vi "FFT_based_prediction_Computationtime.vi"() -> ()   [LabVIEW 2020]
uses:
  <vilib>/Utility/file.llb/Read Delimited Spreadsheet (DBL).vi
panel:
  out "x-y":u32
  out "Time vs Acceleration graph(whole data)  2":cluster{"all rows":dbl[], "all rows":dbl[]}(graph)
  out "Acceleration 3":dbl[](array[numeric])
  out "time 3":dbl[](array[numeric])
  out "array w/ subset deleted 3":dbl[][](array[numeric])
  out "Input vs prediction (zoomed) 2":dbl[][](graph)
  out "truth vs prediction vs error 2":dbl[][](graph)
  out "Input vs prediction  2":dbl[][](graph)
  out "Time vs Acceleration ( Input learning length) 2":cluster{dbl[], dbl[]}[](graph)
  out "magnitude 4":dbl[](array[numeric])
  out "phase 4":dbl[](array[numeric])
  out "ploted signal from each selected frequency 3":dbl[][](graph)
  out "df (Hz) 3":dbl
  out "size(s) 3":i32
  out "xf (frequency) 3":dbl[](array[numeric])
  out "Frequency Interval: delta(f) 3":dbl
  out "Spectrum plot 3":cluster{i32, dbl, "spectrum out":dbl[]}(graph)
  out "truth vs prediction  2":dbl[][](graph)
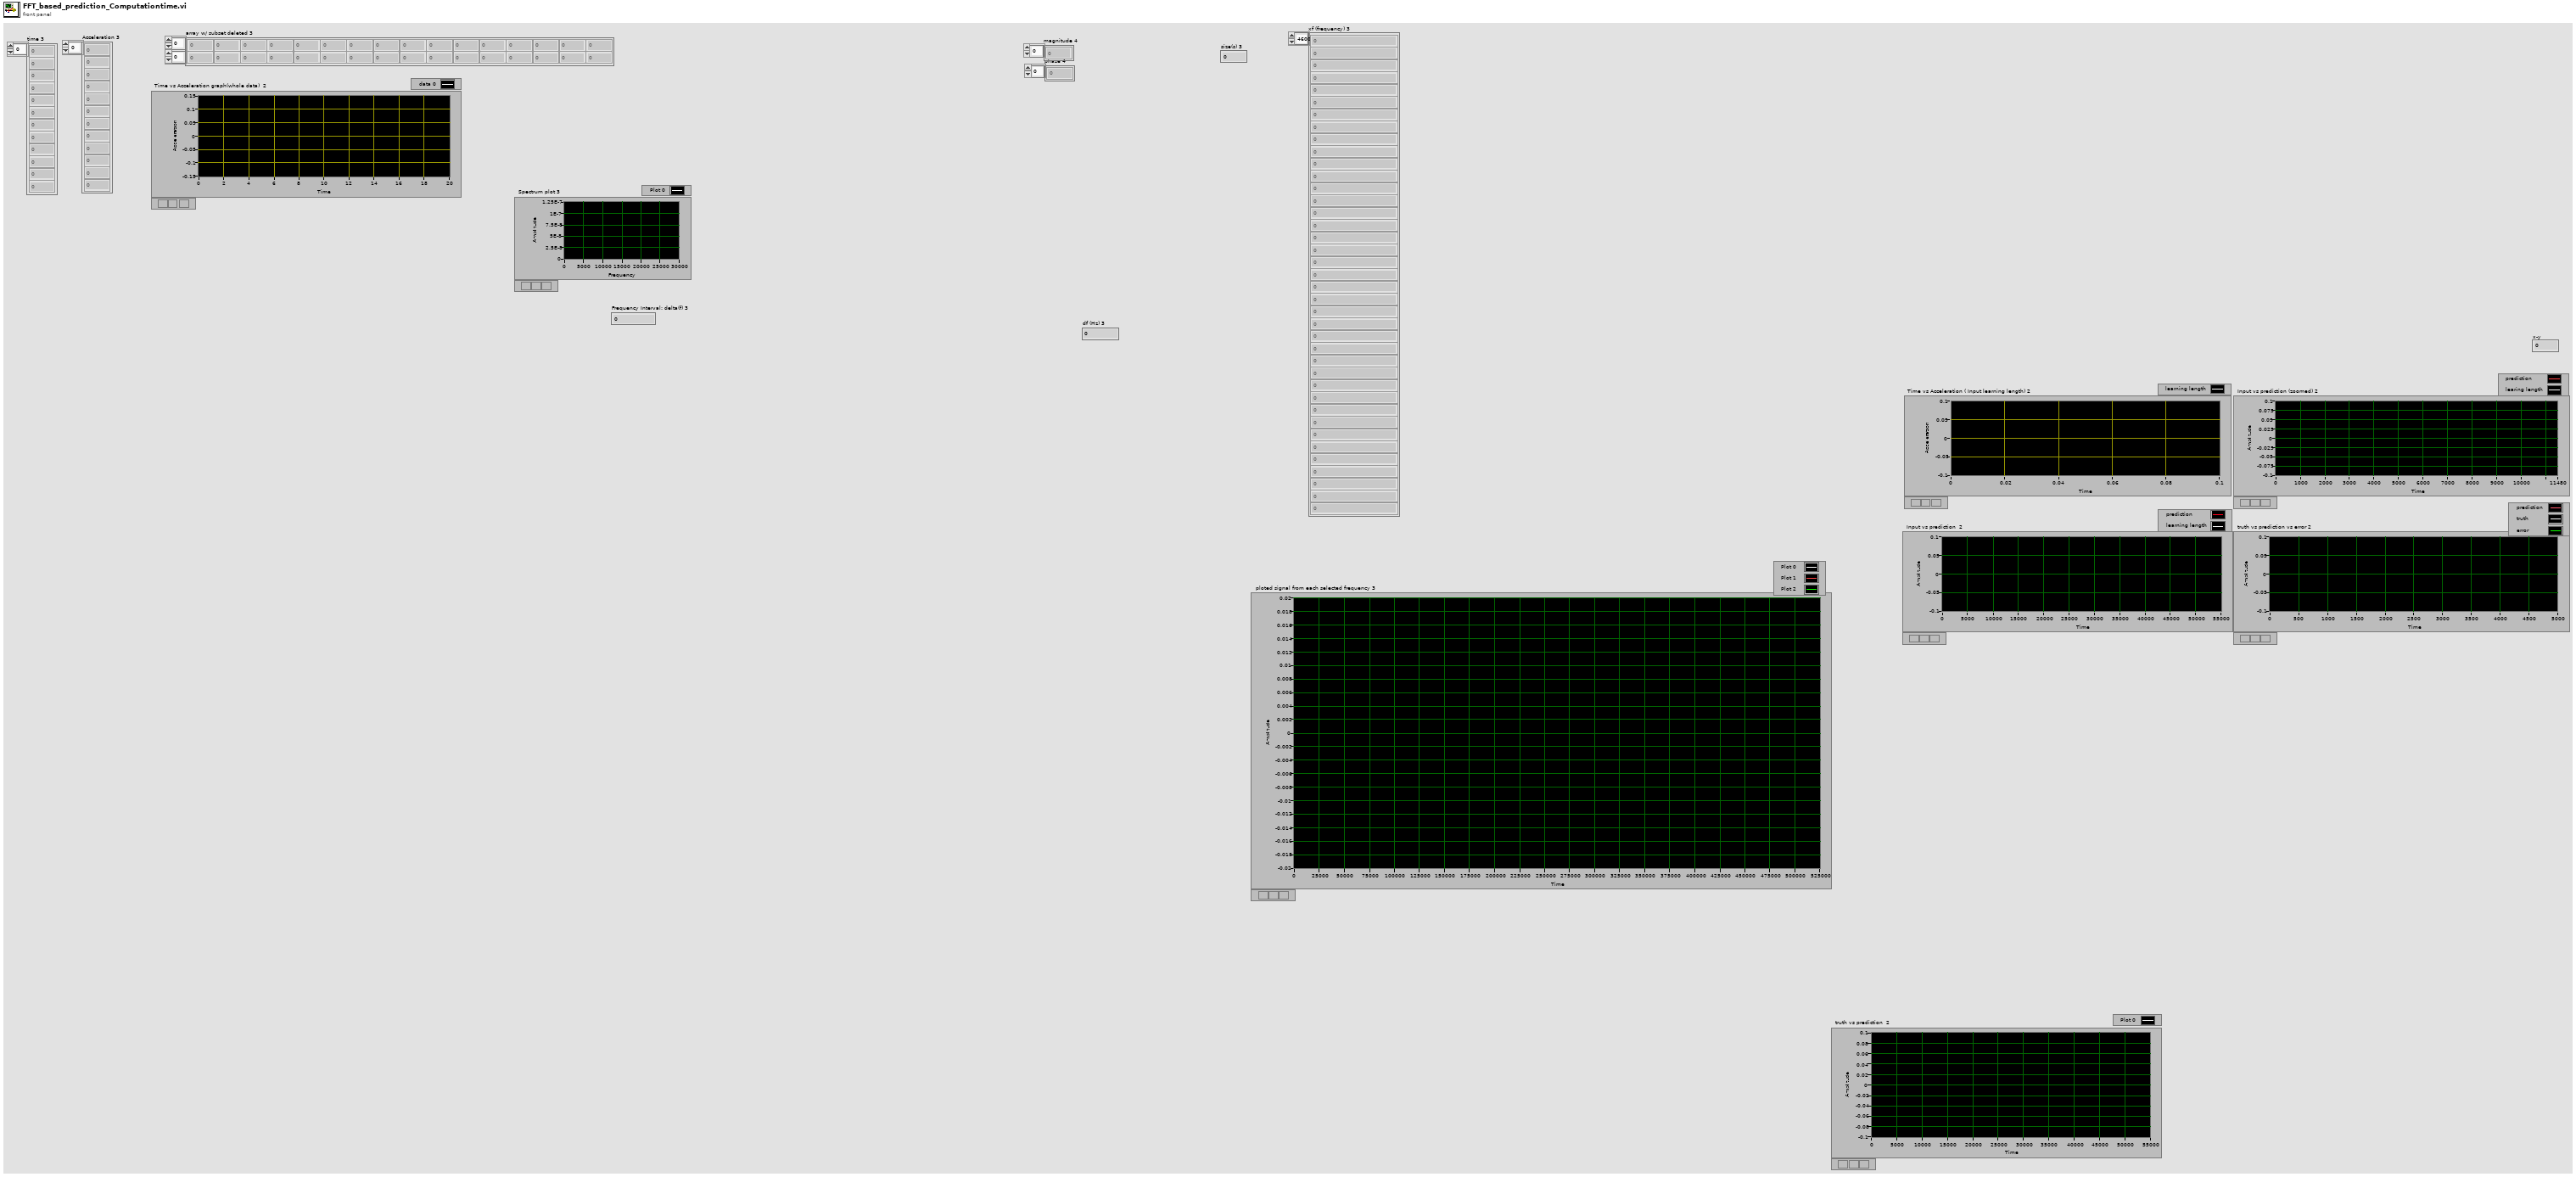
[diagram p1: front panel]
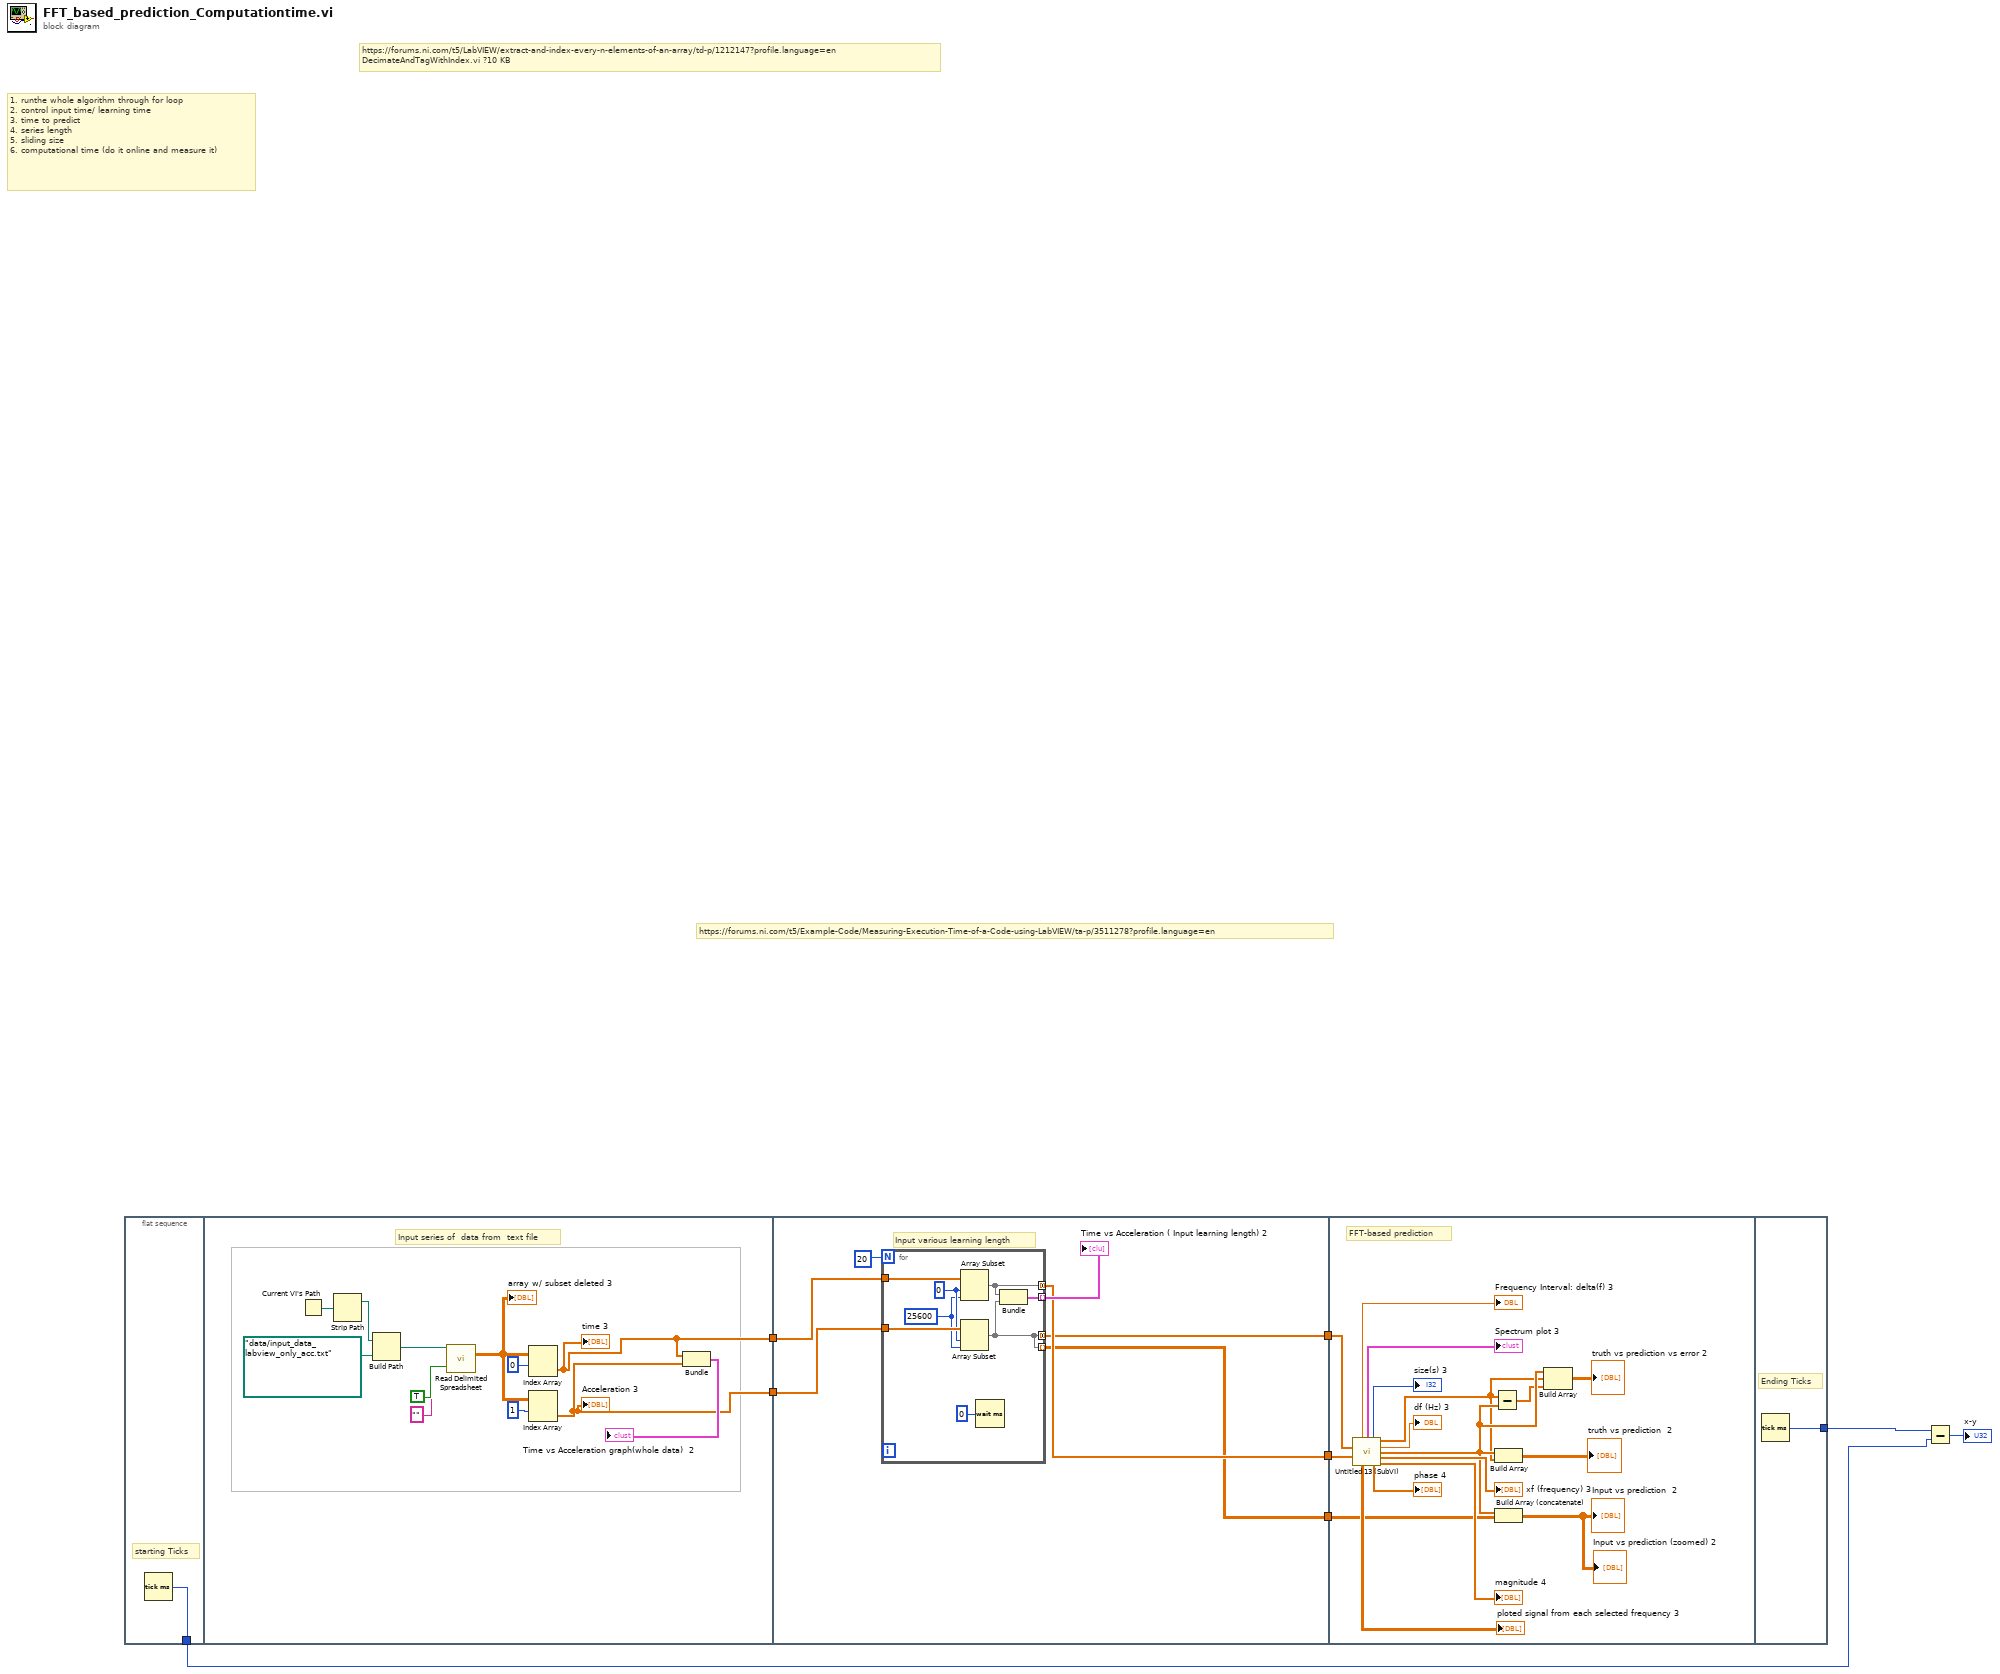
[diagram p0: block diagram]
diagram:
  # "https://forums.ni.com/t5/Example-Code/Measuring-Execution-Time-of-a-Code-using-LabVIEW/ta-p/3511278?profile.language=en"
  # "1. runthe whole algorithm through for loop \n2. control input time/ learning time\n3. time to predict\n4. series length\n5. sliding size\n6. computational time (do it online and measure it)"
  # "https://forums.ni.com/t5/LabVIEW/extract-and-index-every-n-elements-of-an-array/td-p/1212147?profile.language=en\nDecimateAndTagWithIndex.vi ?10 KB"
  n1 = flat-sequence {
    tunnel: [w9] -> w1
    tunnel: [w11] -> w8
    tunnel: [w10] -> w7
    tunnel: w8 -> [w27]
    tunnel: w7 -> [w26]
    tunnel: [w24] -> w6
    tunnel: [w23] -> w5
    tunnel: [w22] -> w4
    tunnel: w6 -> [w39]
    tunnel: w5 -> [w38]
    tunnel: w4 -> [w37]
    tunnel: [w54] -> w3
    frame #0 {
      # "starting Ticks"
      n2 = Tick Count (ms)() -> (millisecond timer value=w9:u32)
    }
    frame #1 {
      # "Input series of  data from  text file"
      n3 = Current VI's Path() -> (path=w19:path)
      n4 = Strip Path(path=w19) -> (stripped path=w20:path)  [unwired: 1 out]
      n5 = Build Path(base path=w20, name or relative path=path "data/input_data_labview_only_acc.txt") -> (appended path=w21:path)
      n6 = call-poly <vilib>:"Read Delimited Spreadsheet.vi"("file path (dialog if empty)"=w21, "transpose? (F)"=TRUE, "delimiter (\\t)"="" ("delimiter (\\t)")) -> ("all rows"=w18:dbl[][])  [unwired: 7 in, 5 out]
      "array w/ subset deleted 3" <- w18
      n7 = Index Array(array=w18, index (row)=0) -> (element=w11:dbl[])  [unwired: 1 in]
      "time 3" <- w11
      n8 = Index Array(array=w18, index (row)=1) -> (element=w10:dbl[])  [unwired: 1 in]
      "Acceleration 3" <- w10
      n9 = Bundle("all rows"=w11, "all rows"=w10) -> (→"Time vs Acceleration graph(whole data)  2":cluster{"all rows":dbl[], "all rows":dbl[]})  [unwired: 1 in]
    }
    frame #2 {
      # "Input various learning length"
      n10 = for {
        N: 20 -> [_]
        tunnel: w27 -> [w36]
        tunnel: [w33] -> w24 mode=concatenating
        tunnel: w26 -> [w35]
        tunnel: [w31] -> w23 mode=concatenating
        tunnel: [w32] -> w25 mode=indexing
        tunnel: [w31] -> w22 mode=indexing
        w34 = 0
        w30 = 25600 ("length")
        n11 = Array Subset(array=w36, index=w34, length=w30) -> (w33:dbl[])
        n12 = Array Subset(array=w35, index=w34, length=w30) -> (w31:dbl[])
        n13 = Wait (ms)(milliseconds to wait=u32 0) -> ()  [unwired: 1 out]
        n14 = Bundle(w33, w31) -> (w32:cluster{dbl[], dbl[]})  [unwired: 1 in]
      }
      "Time vs Acceleration ( Input learning length) 2" <- w25
    }
    frame #3 {
      # "FFT-based prediction"
      n15 = call "Untitled 13 (SubVI).vi"("time"=w39, "acceleration"=w38) -> ("Frequency Interval: delta(f)"=→"Frequency Interval: delta(f) 3":dbl, "Spectrum plot"=→"Spectrum plot 3":cluster{i32, dbl, "spectrum out":dbl[]}, "size(s)"=→"size(s) 3":i32, "all rows"=w43:dbl[], "df (Hz)"=→"df (Hz) 3":dbl, "Array"=w44:dbl[], "xf (frequency)"=→"xf (frequency) 3":dbl[], "ploted signal from each selected frequency"=→"ploted signal from each selected frequency 3":dbl[][], "phase 2"=→"phase 4":dbl[], "magnitude 2"=→"magnitude 4":dbl[])  [unwired: 4 in]
      n16 = Subtract(x=w43, y=w44) -> (x-y=w42:dbl[])
      n17 = Build Array(w44, w43) -> (→"truth vs prediction  2":dbl[][])
      n18 = Build Array (concatenate)(w44, w37) -> (→"Input vs prediction  2" →"Input vs prediction (zoomed) 2":dbl[][])
      n19 = Build Array(w44, w43, w42) -> (→"truth vs prediction vs error 2":dbl[][])
    }
    frame #4 {
      # "Ending Ticks"
      n20 = Tick Count (ms)() -> (millisecond timer value=w54:u32)
    }
  }
  n21 = Subtract(x=w3, y=w1) -> (x-y=→"x-y":u32)
